vi "read_attributes.vi"(8 "error in (no error)":errorcluster, 11 "MeanShift in":refnum<class "MeanShift.lvclass">) -> (0 "error out":errorcluster, 2 "attributes":T1, 3 "MeanShift out":refnum<class "MeanShift.lvclass">)   [LabVIEW 2020, in "MeanShift.lvclass"]
uses:
  MeanShift.lvclass
  Controls/mean_shift_attributes.ctl
  MeanShift.lvclass/MeanShift.ctl
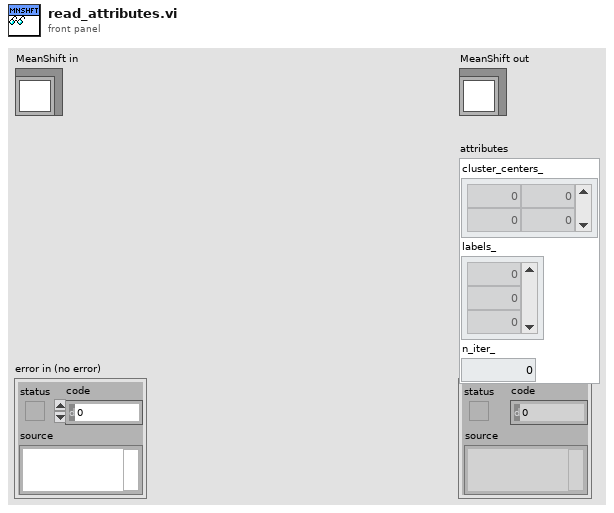
[diagram p1: front panel]
types:
  T1 = typedef "mean_shift_attributes.ctl" = cluster{"cluster_centers_":dbl[][], "labels_":dbl[], "n_iter_":dbl}
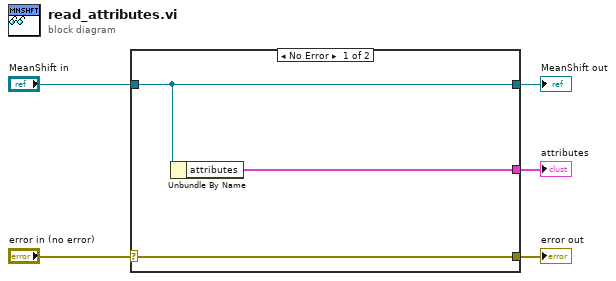
[diagram p0: block diagram]
diagram:
  n1 = case shown="No Error" "error in (no error)" {
    selector: "error in (no error)" -> [w8 w9]
    tunnel: [w8 w9] -> w4
    tunnel: [w7 w10] -> w2
    tunnel: "MeanShift in" -> [w7 w10]
    tunnel: [w6 _] -> w1
    frame No Error {
      n2 = Unbundle By Name(w7) -> ("attributes"=w6:T1)
    }
    frame Error {
    }
  }
  "error out" <- w4
  "MeanShift out" <- w2
  "attributes" <- w1
